vi "NI6071E_RT_ConfigDAQ.vi"(0 "taskID in":u32 format="%x", 7 "NI6071E DAQ Config":T1={"device (1)"=1, "channels (0)"=["0"], "buffer size (1000 scans)"=1000, "[number of buffers] (1)"=1, "measurement mode structure"={"measurement mode"=0, "reserved"=0}, "input limits (no change)"=[], "coupling & input config (no change:0)"=[]} {"measurement mode structure"."measurement mode" items=["no change", "Volts", "Volts RMS", "Ohms", "Diode", "4-wire ohms", "Current", "Current RMS"]; "coupling & input config (no change:0)"."input config (no change:0)" items=["no change", "differential", "ref. single-ended", "non-ref. single-ended", "4-wire"]; "input limits (no change)"."low limit (0.0)" format="%0.2f"; "input limits (no change)"."high limit (0.0)" format="%0.2f"}, 11 "error in (no error)":errorcluster) -> (4 "taskID out":u32 format="%x", 8 "number of channels":i32, 15 "error out":errorcluster)   [LabVIEW 2009]
uses:
  NI6071EConfig.ctl
  NI6071E.lvlib
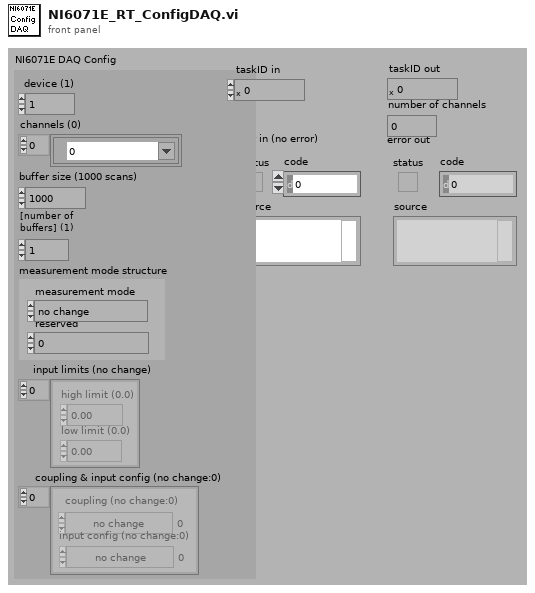
[diagram p1: front panel]
types:
  T1 = typedef "NI6071E.lvlib/NI6071EConfig.ctl" = cluster{"device (1)":i16, "channels (0)":tag[], "buffer size (1000 scans)":i32, "[number of buffers] (1)":i32, "measurement mode structure":cluster{"measurement mode":u16, "reserved":u32}, "input limits (no change)":cluster{"high limit (0.0)":sgl, "low limit (0.0)":sgl}[], "coupling & input config (no change:0)":cluster{"coupling (no change:0)":enum16{"no change", "DC", "AC", "GND", "internal ref."}, "input config (no change:0)":u16}[]}
  T2 = cluster{"coupling (no change:0)":enum16{"no change", "DC", "AC", "GND", "internal ref."}, "input config (no change:0)":u16}[]
  T3 = cluster{"high limit (0.0)":sgl, "low limit (0.0)":sgl}[]
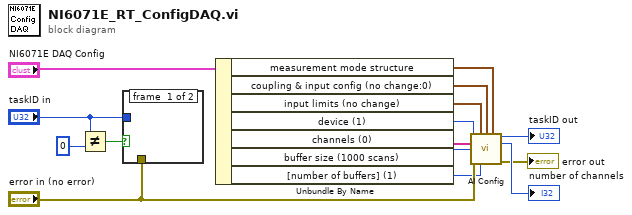
[diagram p0: block diagram]
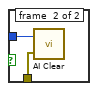
[diagram p2: hidden frame]
diagram:
  n1 = Not Equal?(x="taskID in", y=u32 0 ("taskID in")) -> (x != y?=w4:bool)
  n2 = case shown="True" w4 {
    tunnel: "taskID in" -> [_ w17]
    tunnel: "error in (no error)" -> [_ w16]
    frame #0 {
    }
    frame #1 {
      n3 = call <vilib>:"AI Clear.vi"("error in (no error)"=w16, "taskID in"=w17) -> ()  [unwired: 4 in, 2 out]
    }
  }
  n4 = Unbundle By Name("NI6071E DAQ Config") -> ("measurement mode structure"=w3:cluster{"measurement mode":u16, "reserved":u32}, "coupling & input config (no change:0)"=w8:T2, "input limits (no change)"=w9:T3, "device (1)"=w12:i16, "channels (0)"=w11:tag[], "buffer size (1000 scans)"=w10:i32, "[number of buffers] (1)"=w2:i32)
  n5 = call <vilib>:"AI Config.vi"("device (1)"=w12, "input limits (no change)"=w9, "coupling & input config (no change:0)"=w8, "measurement mode structure"=w3, "channels (0)"=w11, "buffer size (1000 scans)"=w10, "error in (no error)"="error in (no error)", "[number of buffers] (1)"=w2) -> ("taskID"=→"taskID out":u32, "number of channels"=→"number of channels":i32, "error out"=→"error out":errorcluster)  [unwired: 5 in]
